vi "lvBuildSpecAllTargets.vi"() -> (0 "error out":errorcluster)   [LabVIEW 2016, in "lvcommonbuild.lvlib"]
uses:
  lvcommonbuild.lvlib
  <vilib>/Wiresmith Technology/LabVIEW CLI/CLI Class/CLI.lvclass
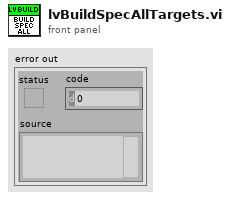
[diagram p1: front panel]
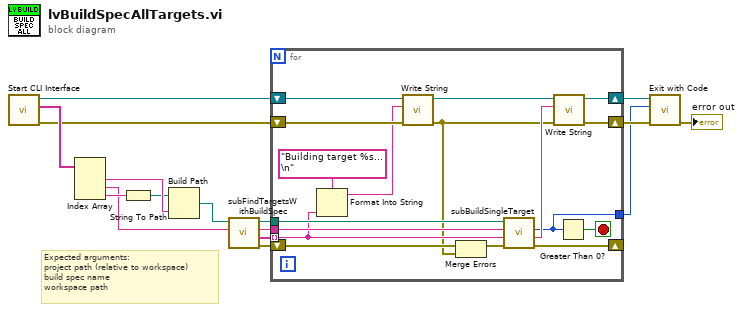
[diagram p0: block diagram]
diagram:
  # "Expected arguments:\nproject path (relative to workspace)\nbuild spec name\nworkspace path"
  n1 = call <vilib>:"Start CLI Interface.vi"() -> ("error out"=w3:errorcluster, "Custom Parameters"=w16:string[], "CLI out"=w5:refnum<class "CLI.lvclass">)  [unwired: 9 in]
  n2 = Index Array(array=w16) -> (element #1=w14:string, element #2=w10:string, element #3=w12:string)  [unwired: 3 in]
  n3 = String To Path(string=w12) -> (path=w13:path)
  n4 = Build Path(base path=w13, name or relative path=w14) -> (appended path=w11:path)
  n5 = call "subFindTargetsWithBuildSpec.vi"("Build Spec Name"=w10, "Project"=w11) -> ("error out"=w9:errorcluster, "Targets with spec name"=w6:string[], "dup Build Spec Name"=w7:string, "dup Project"=w8:path)  [unwired: 6 in]
  n6 = for {
    tunnel: w8 -> [w33]
    tunnel: w7 -> [w32]
    tunnel: w6 -> [w22] mode=indexing
    shift-right: [w31] -> w4
    shift-left: w5 -> [w24]
    shift-right: [w29] -> _
    shift-left: w9 -> [w19]
    shift-right: [w28] -> w2
    shift-left: w3 -> [w25]
    tunnel: [w26] -> w1
    stop <- w27 stop-if-true
    n7 = Format Into String(format string="Building target %s...\n", w22) -> (resulting string=w20:string)  [unwired: 2 in, 1 out]
    n8 = call <vilib>:"Write String.vi"("error in (no error)"=w25, "Text to Write"=w20, "CLI in"=w24) -> ("error out"=w17:errorcluster, "CLI out"=w23:refnum<class "CLI.lvclass">)  [unwired: 7 in]
    n9 = Merge Errors(w19, w17) -> (w18:errorcluster)
    n10 = call "subBuildSingleTarget.vi"("error in (no error)"=w18, "Target"=w22, "Build Spec"=w32, "Project"=w33) -> ("error out"=w29:errorcluster, "Output Message"=w30:string, "Exit Code (0)"=w26:i32)  [unwired: 5 in]
    n11 = call <vilib>:"Write String.vi"("error in (no error)"=w17, "Text to Write"=w30, "CLI in"=w23) -> ("error out"=w28:errorcluster, "CLI out"=w31:refnum<class "CLI.lvclass">)  [unwired: 7 in]
    n12 = Greater Than 0?(x=w26) -> (x > 0?=w27:bool)
  }
  n13 = call <vilib>:"Exit with Code.vi"("error in (no error)"=w2, "Exit Code (0)"=w1, "CLI in"=w4) -> ("error out"=→"error out":errorcluster)  [unwired: 8 in]
